vi "FileGolbalPara.vi"() -> ()   [LabVIEW 2013]
panel:
  in  "UpLdStop":bool
  in  "Len":u32
  in  "MD5":string
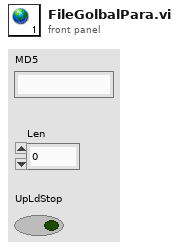
[diagram p1: front panel]
diagram:
